vi "FVIR_Setup_Parameters.vi"(8 "error in (no error)":errorcluster, 11 "UI in":refnum<queue>) -> (0 "error out":errorcluster, 3 "UI out":refnum<queue>)   [LabVIEW 2020]
uses:
  Message Queue/Message Cluster.ctl
  Message Queue/Enqueue Message (Single).vi
  Message Queue/Message Queue.lvlib
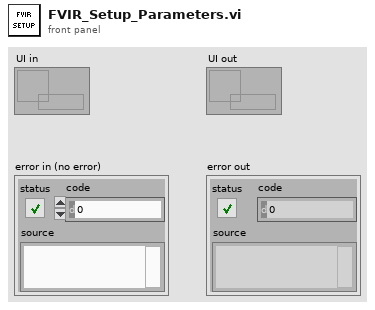
[diagram p1: front panel]
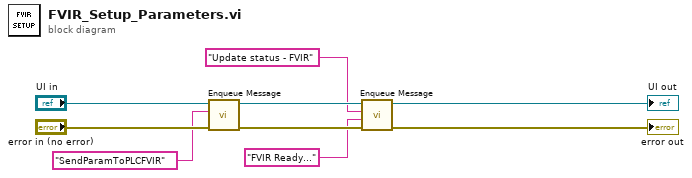
[diagram p0: block diagram]
diagram:
  n1 = call-poly "Enqueue Message.vi"("error in (no error)"="error in (no error)", "Message"="SendParamToPLCFVIR", "Message Queue"="UI in") -> ("error out"=w6:errorcluster, "dup Message Queue"=w7:refnum<queue>)  [unwired: 7 in]
  n2 = call-poly "Enqueue Message.vi"("error in (no error)"=w6, "Message Data"="FVIR Ready..." ("Ready..."), "Message"="Update status - FVIR", "Message Queue"=w7) -> ("error out"=→"error out":errorcluster, "dup Message Queue"=→"UI out":refnum<queue>)  [unwired: 6 in]
